vi "Main_12b-2.vi"() -> ()   [LabVIEW 2023]
uses:
  ENUM_Type.ctl
  <vilib>/Utility/error.llb/Trim Whitespace One-Sided.vi
panel:
  out "Fit Array":i32[](array[numeric])
  out "Stream array":T1[](array[typedef])
  out "Rows Left":i32
  out "Answer":u64
  in  "Puzzle":string="??#.????#???.#?# 1,5,1,1,1\n?##?##??#? 7,1\n??????#???. 1,7\n??#?#??#.?#.??#? 5,1,1,2\n???????.??? 1,3\n?#..##?##??###??#? 2,13\n?.????????.???????? 1,5,1,6\n?.???#???. 2,2\n??#..#???#? 1,1,4\n?.?##?????#??? 1,5,2,1\n.???#?????##??#.? 3,8\n?????????????.#.. 4,3,1\n..#???????.? 4,3,1\n????#??.?.#??? 7,3\n#??#???##??.?? 4,1,3,2\n??#?#?##?.???#??. 6,5\n???.#??.??###?.#?? 3,1,5,2\n?.????##??#?? 6,3\n???..?##????.? 2,3,1\n?.?#????.??#?#.? 1,2,1,3,1\n?.?###.???? 4,2\n?#???..??##? 4,3\n???#????#?. 1,2,3\n#???#???#??#???.? 1,10,1\n???????????????????? 1,5,6,3\n???????#??? 2,6\n??.??.????.?#?????# 1,1,2,1,4,3\n???#???.??#? 1,4,1,1\n???#???##??##? 3,2,3\n????.??????#?.#? 1,1,1,4,2\n?.#??#???? 1,1,5\n??##???#?.##??..? 4,2,4\n??????#.????.# 4,2,1,1\n??????#??#?.??? 2,7,1\n.????????##.?.?.##? 5,2,1,1,2\n.??????????#?#. 3,1,2,1\n?????????????. 2,1,5\n?##????#?.?????.#??? 2,1,2,3,3\n?????????#?.?????#? 1,2,1,3,4,2\n..?.#???.?##.? 1,3,2\n.??????????????? 10,2\n?.?#????#?.??? 1,1,2,2\n??????.#??.?.? 1,1,1\n#???#?#??#????? 1,2,1,5\n???.?.??#????.? 3,6\n.#.???###???.#?..??? 1,8,2,2\n.???.??#????# 2,4,1\n.????#?#?? 3,3,1\n?###??#??## 4,2,2\n??#?#???#???.??. 3,5,1\n???####??##..?#.#.?? 9,2,1,1\n??#?#???#.?. 5,1\n???#????#???##?# 2,3,3,1\n?#???????#???#??? 1,3,3,3,1\n#???#????#.##..? 8,1,2\n?????.?#?#??? 1,5\n.??#.??#?.? 1,1,1\n?#?#???#???.??? 1,1,4,1,3\n.????#.?.#??? 1,1,2,1\n.??#?.??#? 4,2\n#????????. 1,4,1\n??.#?#????#?...?? 1,8,2\n?#.#?#.??##? 2,3,1,2\n...??.?#?? 1,1\n?.?.????#..? 1,2,1\n?##????????.??.?#??? 6,1,1,4\n?.??#.??.?.???? 3,2\n.????.?????.???.?? 4,1,1,3,1\n?????????##???????#? 2,1,1,2,2,2\n???.?????.????? 2,3,5\n???#??????.??#??.? 1,6,1,1,1\n??##??????###??? 12,1\n?.??.?????? 1,1,2\n??#??????#?.. 2,5\n???#####????. 1,8\n.?#?##??????#??.???? 6,2,1\n?.#??#???????#????? 1,1,12,1\n??????????#.?..?##? 1,1,1,1,3,3\n???????#???.??## 10,4\n.?#????.?.???..? 1,1,2\n.???#?#????? 2,2,1\n#????#?.????##?#?# 1,5,1,5,1\n???.##??????##??#? 1,2,8,2\n??#????????????#? 6,7\n????.??.#.?#?#? 1,1,1,1,4\n??##?#??.#???? 6,1,4\n?#?.?#????????#?. 3,2,4,3\n..??????##?# 2,1,2,1\n?????????.???? 4,1,1,1\n.??#?????.?.?. 1,6,1\n#.?#?#??????#??# 1,6,2,1,1\n.#?.#.##??# 1,1,5\n??#?????#?????? 5,4\n.#??.?.?.? 2,1\n.?#???##.????##?? 7,2\n?#?.??????#??????# 1,8,3\n?.#??#??.?#.. 4,1,1\n?#?#?#??????? 7,1,1\n?#???????? 6,1\n????#..?#???##? 1,1,2,3\n..?????#?###??.? 1,9,1\n?##???.???#?# 4,4\n??.??#???..??#? 1,2,1,3\n#?#??????.??#?? 8,1,3\n???#?##?#?? 2,6\n.?.???#???.#?????? 1,3,1,5,1\n?#.???????# 2,2,1\n?.???.??.? 1,1,1\n?#?#?#??????#??#??? 1,5,2,4,2\n?#??.?#?????.?#. 4,6,2\n#???.?#?#??#?.??#? 2,7,1\n.??#...???????. 3,1,1\n?..???##??. 1,6\n??#??#?#??? 2,4\n?.?.??.??????#?. 1,7\n?.?????????.??. 2,2,2\n???.?????? 2,1\n???.??????????? 1,3,4,1\n?#????#???#??? 10,1\n??#???.?????#???# 6,3,1\n????.?##??#??# 3,8\n?????????????. 1,7,1\n?..?????.#???.. 1,4,2\n?.???#???#? 1,5,1\n#???.????? 2,1,1\n?#.??#?.???? 1,1,1,1\n????.?#???.???. 1,1,4,2\n.?#??#??.??????? 2,4,6\n.??.?##.??#?#.??? 2,3,2,1,1\n..??????#?.?? 2,2\n???#?#??.##. 3,2,2\n?..?????????##?#??? 1,13,1\n??#?????#?.??#?????? 6,2,5,2\n???.???#???# 1,1,3,1\n??##????.?. 4,1\n??#??#??#?. 3,6\n.??????#????#.#.?? 1,1,8,1,1\n?#?#?.?.?.###??#???? 5,1,1,3,1,1\n???.#?#???.?? 1,1,5,1\n?????####??????? 2,5,2,1\n????.??#??#? 1,1,2,1\n??.?????#?#.????? 2,3,3\n?#??#?#?.????.??? 2,3,2,2\n?????????#??.??????. 1,6,1,1,1,1\n???.##?##??#? 1,6,1\n????#?.??.. 4,1\n?#??#?#???.????#?# 4,4,6\n?????#??#.#? 1,2,2,1\n?#?#?#??###??? 1,1,7\n.##?.????? 3,3\n??#???###????? 1,6\n.?###????????##?#?? 7,1,5\n..?#????????#? 3,5\n#?#???.??? 1,1,1\n#???????????#??.??? 10,3,1\n???##??#??#?.?????. 10,3\n?#?????.???????## 3,2,5,3\n??.??#####???. 2,8\n???.?????? 1,1,3\n???#???????????. 6,4\n#???#?????##???.?#? 2,1,1,5,2\n?#?..???#??????. 2,7,2\n?????##?#? 2,3,2\n.#?..????# 2,3\n???????#??#.?..??.. 3,1,1,2,1,1\n?.#??#????? 1,3,2\n???..?.?.? 1,1,1\n?#.?#??#???.##.? 1,1,4,2\n???#?#.??#??? 4,1\n??????#????.???? 6,1,1,1,2\n???..??.#???? 1,1,1,2\n????????.? 1,1,1\n?..#??.??. 3,1\n?##.??#??? 2,1,1\n?????#?????#?#?? 2,12\n?#??????#???.?? 1,6,2,1\n#??.???.??##???.#? 2,3,7,2\n???????..????#????? 2,1,1,7,1\n????#??.?????? 1,2,4\n?###?#?##?##??.??. 12,1\n?#??#.?.??#?... 3,1,1,1,2\n??#??#??#????#? 9,2\n???????##????? 1,1,5\n?.?#????#?.??.?? 3,3,1,1\n???..??????#..??#? 1,1,7,1,1\n??.???###???#..? 1,1,5,1,1\n??.??.#????#????# 2,1,7,2\n??????#?#??????# 1,6,1\n#?.?...??.??????? 1,1,1,6\n??#?##??#?..## 7,2\n?#?###..?.#?##??.?.# 5,6,1\n.??.?.???. 2,1,1\n?.???..?.?#?.??.???? 1,3\n.#?.??????.?.?#??? 2,6,4\n???##...??. 3,1\n????????????#?????. 4,6\n????#.??#? 1,1,1\n?.?#.??..??#?????..? 1,2,1,8\n?????.??.? 1,2,1\n??????##?.?? 1,4\n???.????#??? 1,1,5\n.??#???.#.#??#??. 6,1,2,1,1\n?.????#??##?????? 1,1,1,7\n??????##.??? 3,2,1\n?.????#?????.?.? 1,4,2,1\n?????????????## 1,1,2,4\n.?##??#??.??# 4,1,3\n??#?##??#?? 2,5,1\n?????.###??.?.#??# 1,1,4,1,1,1\n.????????##?#? 1,7\n??????????.? 7,1\n.?????###????..#. 12,1\n????.????? 3,1,1\n#.??#????#????#????? 1,5,1,7,1\n.##??????.??##? 7,3\n?..?.???#?????###? 1,1,5,5\n??????#???. 1,1,3\n??.#???????##????. 1,2,3,6\n?.?.?.?.#???????#?. 1,1,1,1,2,7\n?????#????????. 1,1,1,4,1\n?.??#??#?? 1,1,2\n??#???.#.?#?#?? 1,1,1,1,5\n?????????.? 4,1\n??.?????#?.?.#?? 7,1\n??.?#.?????#??. 2,7\n?????##..? 1,4\n?????????. 4,1\n??.?..?#???? 2,3,2\n????.####??###? 2,4,4\n?####???##??????? 10,1,1\n???#?#???# 1,5,1\n????###.??.?????#??. 6,1,6\n#???????#?. 2,1,4\n?#?.???##???????#? 3,1,2,1,6\n???#??#?.?.?????? 1,5,1,1,4\n?.#???##???.?.## 1,3,2,2\n???..##?.?.? 2,2,1\n?.#?#?????. 3,1\n????.##?#?#??##?? 3,12\n#?##???????? 1,3,3,1\n???.#?.????##? 1,2,1,4\n???.??#???? 1,3\n.???###??.???????# 7,5,1\n?#.??.?#???##?. 1,1,1,4\n.????###????? 2,6\n???#???.???????#?? 1,2,1,3,4,1\n.?.?????????? 3,5\n??#???#?.###????.?? 7,3,1,1,1\n#??###??#?#.????? 11,1\n#.?????#??#.##???.? 1,1,7,5\n??????.????#???? 1,1,4,1,1\n?.?#?#?#??###?? 7,4\n????#???#?#?###????? 1,2,10,1\n????#????? 1,4,2\n???.#??#????.?#??.?. 3,2,1,1,4,1\n?????.?#??????. 1,2,1,1,1\n?#???????#?#?#???.? 2,12\n?#??..??.???###?? 4,2,1,5\n##????????#.? 5,2\n#?#?.?.??###??#?. 4,8\n??##?.???? 3,4\n?.????##???????? 8,1,1\n#????#??#???#?#.??? 15,1\n?.?????.#? 4,2\n?.##???..?? 1,3,1\n#????#??????????#?? 2,7,2,3\n???.????#? 1,1,2\n??..#?????### 1,3\n????????.?? 2,4,1\n#??##??#.?????.??? 1,5,2,1,1,1\n???#.?#?#?. 3,1,2\n?##?#??????#?#.# 3,3,3,1,1\n??.#?..??? 1,1,1\n?#??.???#? 1,1,3\n???#???????.??##?? 8,3\n??.#.?#???#??.? 2,1,7\n??????.####?.?#?# 4,4,4\n??????????? 2,2,1\n?#?.??.???.? 2,2\n????#?#?## 6,2\n.??###??????.? 5,3\n.???#.#????? 3,5\n?##?#?.?#?#??. 6,2,1,1\n#.???.??#?####?..? 1,1,1,8,1\n????#???#???# 1,1,2,3\n?????.??.#???#? 3,5\n?#??..?????????#?. 1,1,3,1,4\n#?????????????.?? 6,1,1,1\n?#?????..?????#??# 3,1,1,5\n???????.???????????? 1,4,1,9\n.????????????.. 2,1,6\n.?#??????. 2,4\n??#??#???#.???#? 1,5,2,1,2\n.?.???????.?.#??? 4,1,2\n##?.??##?..???. 3,4,3\n??..??#??#?. 1,6\n??#??????????##???? 2,6,4,1\n??..????##?????? 1,5\n##????????.??.#??? 2,6,4\n?#??#...?????# 2,2,1,2\n?..??????.???.?# 1,1,3,1,1\n.?###??#???#???? 7,4,1\n?#?.?????. 2,2\n??..????.?????# 1,1,2,2\n??##.#??????.##??#?? 1,2,1,1,1,5\n??.##??????#???#??? 4,8\n??#?????????. 4,3,2\n#????.???? 1,1,1\n?..??.?????? 2,3\n??????#??###???? 1,1,9,1\n?????#?#???????.. 1,6,3\n?#??.???#?##. 3,3,2\n?..##?#???????#?? 9,1\n???.?#?#?#?. 1,5\n???##?#???#?# 8,3\n?##??#??.??.???????? 2,3,1,6\n.??...?????????#.#? 1,6,2,2\n????.#??#?#.##?. 1,1,1,3,3\n?#?#?????.??????. 5,3\n??.????##???. 1,5\n????#?.???? 2,1\n????..??#???. 4,2,1\n???????.?# 2,1\n????????????? 1,1,3\n???##??????###.?#? 2,2,2,3,1\n??????#?#?#?#?## 3,10\n?????#??..????????? 8,5\n??##???????.??? 6,1,1,2\n?.???.????.??? 3,1,1,3\n.?.???.??? 1,2\n.???###???#??.?? 5,1,1,1\n????#?.##?###.# 1,3,2,3,1\n.?#???????? 1,4\n?#?#?????????### 8,6\n?????..???.???? 4,3,1,1\n..?#?.?#??? 1,5\n.????.??#? 3,3\n?##????.?#??????..?? 7,3,3,1\n?????##??.?.??...?? 9,2,2\n??..#??####??.?.?#? 8,2\n??????##????? 1,1,6\n??????#??.???#? 7,5\n???#..??.????. 4,1,2\n.#?.?###??? 1,4\n????###?...?#?#? 8,4\n?????#???#??????? 1,1,6,1,1\n.??#?#?##??????? 7,1,1\n.#.?????#.?#### 1,2,1,1,5\n?#??..#??.#?? 3,1,1,1\n????#??.???. 3,1,3\n#.???#???. 1,2\n???.???##.???.? 1,1,2,2\n?#?#..?#????##?.?. 3,9\n.?.??.????? 2,2\n??????.?.##?#?.? 5,4\n???#???.????? 7,1\n??####?????.???#?? 6,3,4\n?.?...?#.#?#??? 1,2,5\n??.??#??#?#?#??.?? 2,3,7,1\n?#?.???????? 1,1,1\n????????#?##?#??? 1,2,9,1\n#???.???#????.??#??? 3,1,1,1,4,1\n.??#?.?.#??? 2,1,2,1\n.?##?###.###?#?.??. 6,5,2\n.?.???????#????##? 3,10\n?.##???..#? 5,2\n????????????#??.???? 1,1,10,1\n??##??#.??#??#?? 5,3,2,1\n?#???#.??????..# 6,4,1,1\n????????.? 1,2,2\n?????#??#??#????#??? 14,2,1\n???#??.???#?#???? 4,7,1\n.?.##?.???#??..????? 1,3,4,2\n??????#??????? 1,1\n..#?##??.????. 5,3\n??????????#.? 4,1\n#????.???.? 1,1\n.?..?#.??? 2,1\n?#.??##??.##?.?? 2,4,2,2\n??#????#??????? 9,1\n.#?.##?##.#???? 1,5,1,1\n?#?###???#??#?.??? 11,1,1\n???#??..?? 3,1\n#?#??????#?????#? 12,2\n??#?#?.???.? 2,2,3,1\n?#???.?.??#?#???? 5,1,8\n.???#?#??#?????. 10,1\n??????.?????.? 5,1,1,1\n.?.??????????# 3,7\n.#?.??..##??.?#..#? 1,1,4,2,1\n?##?#??.??###?????# 2,1,1,1,7,1\n?##?.???.? 2,1,1\n?????#.#?##.?#? 1,1,4,1\n?#?.??.?#.#.##.? 2,1,1,1,2\n???????.#.??##??.?. 6,1,3,1,1\n.?#??#???????#???.#. 3,1,1,2,4,1\n?????#?.##??##??.?? 1,2,2,3,2\n#??.???????? 1,1,1,1\n????#?.##?.?#?#?# 5,2,5\n.?.??.#?????????..?# 1,1,6,1,2\n???#?#?????. 7,2\n???????##??#?.?#?.? 1,8,3\n.?..?#?#???? 4,1\n??.?#??.????. 1,1,3\n????##???##???#??? 12,4\n?###?#??..#?.??? 6,1,2,1\n##??..##?#????# 3,2,1,1\n?????#?##??##???#?? 2,13\n#?..???##???##?#???? 2,6,4,1,1\n.????.?....#????. 1,3\n?.?.??#??#.?# 1,2,1,2\n???#??.??#.? 1,1,1,2\n.????#?#???#??????? 12,1,1\n?..#??#?##??#???? 1,1,2,3,5\n.#??##?##??????.?# 2,11,2\n.?.#?#?.?#???#.? 1,4,6\n?#.##??.????? 2,4,4\n???.??????.??. 2,1,1,2\n???????.?##.#???.? 1,1,1,2,3,1\n??..???????#?.? 5,2\n?????#????? 3,2,2\n.##????..#??.. 6,2\n????.??????.???###? 3,3,1,5\n??????#?.???# 1,3,1,1\n????#????. 6,1\n??.?#????. 1,4\n??????#???##???. 6,1,3,1\n?.?#.????. 1,1,4\n?##??.#?#??.#?? 3,1,1,1,1\n?.?#??????. 1,5,1\n???????#?. 1,4\n???#????#?##?#?????? 2,2,1,1,6,1\n??##.?????##??#.? 1,2,7,1\n????????.# 4,1\n.???#????? 1,1,1\n?.?#??.????.?#?? 1,4,2,2,1\n.?##?#???.??..?#? 3,3,3\n?#??.?.?#??? 1,1,4\n????..#????#.?? 1,1,1,3,2\n???#?..??? 5,1\n?##???##.?. 3,2,1\n??#???.???### 2,1,1,3\n????.?#??##?. 2,2,2\n?#???##??#?????#.??? 2,11,1\n???#??..?##??# 5,6\n????.??#???.#?#.?#?# 2,5,1,1,1,1\n?.??????#??? 2,3,2\n#.#???..????????. 1,1,2,6,1\n?.?..?.#??????##?? 1,1,1,1,3,5\n.??.?.???? 1,1,4\n#??#.?#?#???#??????# 1,1,2,1,1,8\n?????.?#..#. 3,1,1\n????##???.?????.. 5,3\n.????#???????? 1,5,1,1\n##?..#.???#?????? 3,1,1,2,1\n#??##???????????. 1,11,1\n????????#. 2,1,2\n.#?#?????????. 1,4,2,1\n#??#??.????????????. 5,5,2\n..?#?#???#???????.?. 9,1,1,1\n?#?.?????????... 1,6\n??###??#?#?.? 5,2,1,1\n.?????????.??... 6,1\n?.?.#??#??????#?#. 1,2,7\n??.?#?.#??.??. 1,2,2,2\n?##?#.?#?. 3,1,1\n??.??####???... 2,6\n.?????#????..?..??## 7,1,3\n.#?##???.? 5,1\n?.?.???#.???. 1,1,2,1\n?????.???## 1,3,2\n.????#??.??.?. 5,1\n.?#??.???? 2,4\n??#?.??#?? 2,2\n?.??.??????.?????? 1,1,2,1,1,5\n?????#??????.??? 1,5,2\n#..?#??.?# 1,2,1\n???????#???#?#???.? 5,8\n??.?#??#?? 1,2\n????#.#??#? 3,1,1\n#?#?..?..?????#??? 4,1,2\n??????.?##?##.??? 1,4,6,1\n?.????###??? 1,8\n??##???????##?????. 8,4,1\n?#.?#.?.?????? 1,1,1,6\n???#?.?.#??##???##? 2,10\n.?????#?.?##????#?# 1,3,2,5\n#?.?.?#?..???#? 2,1,1,2,2\n..???#??.??#?? 5,3\n.????##??? 7,1\n??#?###???# 7,1\n?????????????????. 10,5\n??#?#?????????###?? 3,1,1,1,4,1\n????##???.#??? 1,6,1,1\n.##??????##?..??#?## 11,2,2\n?#.????????? 2,1,1,2\n??????#?.??#??..???. 3,1,5,3\n.?##??????????#???? 3,1,1,1,2,1\n?#?...?#?????#?.? 2,8\n###?#.#?#?????.#???? 5,1,2,2,4\n?.???#?#.?????#?.? 6,5\n#????#???#???#?#? 2,2,3,3\n??#??.??#.?#? 2,1,1,2\n##.?...????????#?#? 2,9\n??#?#???#???? 4,1,1,1\n.???#?.?????.?#?.#. 4,1,1,1,1\n??#.?????#?????##? 1,1,1,7\n#???????#?????#? 1,1,8\n????##?#?#??##???#?. 1,8,6\n#.???.?????.#?? 1,1,2,3\n##?????#??.????#? 2,1,3,6\n#???###?##.? 1,4,2\n#..??????#???.. 1,10\n?????#???.?#?#??# 7,7\n???.#????#?????.#? 1,1,1,6,1,1\n??.#?#?????????.?# 1,4,2,2,1\n?#?#?..?#? 1,2,2\n?.?##.???###?? 3,5\n.?#????#??..?? 2,5\n???#.#??.?.????..#?? 2,3,4,1,1\n???#..?????.? 1,1,5,1\n?##?#??????##? 4,1,5\n??#.#?###?##?????#? 1,1,8,1,1\n.#?#??#.#?.? 1,1,1,1\n????????#?#?##??# 5,1,1,5\n.??#?.?#?????.?????? 3,7,4\n?#?????#.?#? 2,5,2\n????.?#????#?????#? 1,9,2\n?#????#???.??.??.. 7,2,2\n?#.##???????.?#.? 2,5,1,2,1\n?.##?#?.????#?#??. 2,1,6\n?###??#.#????##.?? 5,1,1,1,3,1\n.??#?????#???#?.# 3,1,2,2,1\n?.????.??.#?????? 1,3,1,5,1\n????##?##?? 6,3\n.?#???.?.????? 2,1,4\n?????...??.. 1,1\n??#????..??# 1,2,2,3\n?###.?????#.???#? 4,3,1,2\n???##????.?#.?#??? 1,2,2,2,5\n?#.?????.?###?##??.? 2,5,6,1,1\n.????.??.?????????? 3,10\n??.?#?#.#..??? 1,3,1,1\n?.?#?#??.?. 5,1\n???#.?????##???#??? 2,13\n??#???#.#???#???#?? 2,2,11\n?#???????? 4,1\n??????##???##????# 2,10,1\n???#????#?? 3,1\n##????#.?.? 3,2\n.????#?????? 6,1\n?.??.????#? 1,4\n?????????.? 1,4\n#?#??#?##????#????#? 14,3\n#..#????#??? 1,1,4,1\n.?.##????.?? 1,2,1,2\n???.#??#?#?.?????? 1,1,7,1,1,1\n..?#????.#???##????? 3,2,7\n?????.??.? 3,1\n.?#??#?#..?#?.?##.?? 2,4,2,3,1\n???#?????.# 8,1\n????..##?.??#? 1,2,3\n.?????.?#? 1,1,1\n??#?.#?#?#?.###?. 1,5,4\n???.#????##.???##? 1,3,3,5\n?????????#?#?????? 7,2,1,1,1\n#.?##.???.?#?..?.#. 1,2,1,2,1,1\n???#.???.?? 1,1,3\n??.?.??###??.????.? 1,1,7,1,1,1\n.?.#.?#?##?.???# 1,1,5,1,1\n???###?#???# 8,2\n?.????.#..##??? 1,1,2,1,4\n??#????####???#?. 3,8\n#..?#????##?#?. 1,3,3,2\n###.??.##.? 3,1,2\n???##?.????#?#??? 4,5\n?.??.?.?.??? 1,1,1,1\n.#???##??#???##???? 1,1,5,4,1,1\n?..##..??#...?.?.?? 2,1\n?#..#???.?.??# 2,2,1,1\n????#?.#??.? 1,3,1,1\n?#?????#???.????? 3,3,1,2\n#.????###???.?#???? 1,7,2,2,2\n?????.?????? 3,1\n.??#???????. 3,1\n?.?#??.?#???##?#?? 1,1,1,11\n?#????#?#. 4,1,1\n..#?###???#.??? 1,7,2\n#....????? 1,1,1\n?.????????.? 4,1\n##?.??????.#??? 3,2,1,1,1\n?????.?#.?????#??.. 2,3\n?#??##?#?#?.??##? 7,2,3\n.?.?????##.??? 1,2\n.#?##?##?.?????.?#.. 7,1,1,2\n???..???#?. 1,1,2\n...?.???#?#? 1,4\n?????#????#.? 7,2\n??#????##???##. 3,2,4\n???.???????. 2,1,1,1\n###?..?????.. 3,4\n.???????????..?. 4,2,1\n?.?.#??.?? 1,1,1\n?????????????#?? 6,6\n..#?????.??? 4,1\n???#??#?##.?#?.?? 7,3\n#???###??????#?? 1,1,3,2,3\n?##??.??#??????#???# 3,9,1\n???#??#??.??????#??? 7,3,1\n.???###??##?#.?.??? 6,2,1,2\n?.?#?#?.?.?#? 3,2\n.??#.?###???##?? 2,5,3\n????.?????#??###?? 3,12\n?#?##?#..#??#?? 5,1,1,2\n??#??...???#?#???. 1,7\n???##???.???#.?. 7,3\n??.#???#.# 1,5,1\n??###???????????# 5,4,3\n#??..#??##.?????.? 1,1,5,2,1,1\n????#.???#????.. 3,4\n#?????.#??? 3,2,3\n?#?.???????. 2,2,2\n?.?????????## 1,1,4,3\n#????????..#?#????? 3,1,1,3,4\n???#??#??????????.. 7,1,1,2\n?##.??###???#?#??# 2,1,3,1,3,1\n?#?.???#?#?#?.??# 3,5,2\n??#????.??#?#? 3,3,4\n###?##???#?#??.?.# 8,3,1,1\n.??.?#???#??? 2,1,3\n.???#??###?? 1,6\n???????.???????? 7,1,2,1\n.??###?.??#.? 5,3\n?#???#???????#?#???? 2,5,1,4,2\n????.?????#?????? 1,1,7\n.??.?.?#?##?#???#?? 1,11\n?????#???? 5,2\n?.??.???.#?? 1,1,3\n????#???????? 5,3,1\n#?##????#???#?.?#.# 4,3,1,1,1\n??#??????#?? 1,1,1,4\n.????.#?????#?? 1,2,1,1,3\n????????????????? 1,4,3,2\n????.#?.##?##?#?#?? 3,1,5,3\n??#?###??? 1,3,1\n????#???....? 8,1\n.????.???.???..???. 2,3\n?????.??#? 4,2\n#??.#.????#.???###? 2,1,1,1,1,4\n.???????.??????# 6,5,1\n??#??#?????.??#. 1,4,1,2\n??#?.??.??????#?#??? 4,1,3,1,5\n?#??#???????#..??? 4,7,1\n???#?##?????.?? 5,2,1\n.?###?????#?##??. 6,7\n#??#..??????#?? 1,1,7\n.??#?#??????# 4,1,2\n.###??####????#???# 4,13\n????#?????.?. 6,1\n#?##???#????? 5,1,2\n??#?.##??????????? 4,4,5,1\n.????#???? 2,1,3\n?.?#.???????#?.????. 2,4,1,1,3\n?.?#?????##??????? 2,10,2\n?????..???##? 2,3\n?#.#.???#???.? 1,1,1,4\n.?##???##?????###??? 15,2\n?#.#?.????.??.?#?.? 1,2,3,1,1,1\n????#??????. 5,1\n?.#.????##??.?. 1,7\n??.?#?..??#?????.? 2,6\n???##?.#?.?#? 3,2,2\n?#?.???.?? 1,2\n?????????..?#??? 1,1,2,2,1\n?#.??..??? 1,1,2\n??.????##???? 1,1,3,1\n??####??????#.?.??? 5,1,1,1,1,1\n.??#????.?# 2,1,2\n..#?#???##???.?.??# 1,1,4,1,3\n??.##..??. 1,2,2\n?#???#?????? 2,5\n????##?#?.???.? 5,1\n.?#?..????#??.??? 1,4,1\n.#####??????#??. 7,5\n???.?.?.##?#???. 1,5\n????###??.????#?? 8,5\n?????#.???#?.?.?# 4,4,1,1\n????????.?###????#? 1,3,4,1,3\n?.?????.?#?????# 1,3,1,2,1\n??.??????????? 1,3,1,1\n???.?????#??? 1,6\n?##???#?#????#????#. 3,3,3,2\n??#?.?.???### 2,1,3\n#??..?##??????.??? 1,1,3,1,1,1\n???#??.?.#???#? 6,1,2\n?#?..????? 3,2\n?##??#???? 5,2\n??.??????.?#? 1,4,2\n.#?##???.???#??????? 7,4,1\n?.#???..????? 4,3\n.???..?#??##?? 1,7\n.#???????.??? 1,1,1,2\n?#?#???????##. 6,3\n#.?.#?????#??#?#???. 1,1,1,6,4,1\n.???????.?#?#??????? 2,5\n??.?.?????? 2,3\n???.????..#? 1,1,1,2\n??#??.?#?..???##??## 2,3,8\n#??.?.?#??#?. 2,5\n?.????.????????? 1,2,3,1,1\n???.??.??????????#. 1,1,1,3,3\n???????.??? 1,1\n##??#????????.?????# 2,2,6,1,3\n??.?????##????## 2,1,1,8\n???.??#?????#??.. 1,3,6\n??#?#??#???????.? 7,1\n.?#.????#??#? 2,4,2\n?????.??#.??? 1,2,2,1\n??##???.????????. 6,6\n..???..?.?.? 3,1\n??#?.??????.. 2,1\n???????##?????. 1,1,4,2,1\n??##..??#???. 2,4\n?????#??????#? 1,2,4\n..??#???#?????#?? 3,2,5\n???.??#??.???#?#??? 2,5,6,1\n?#?#.??##.?. 3,3\n#??#.?????.?? 4,2,1\n?#???.?#???#???.. 4,9\n????.??????#?#??# 2,7\n??#.??????????????? 3,7,5\n??#????###? 1,4\n???#????#.#.??.. 1,3,2,1,1\n???#?.???? 1,2\n?.??.?#??? 1,3\n??.????#??#.?.? 1,2,1,1,1\n..??????.?? 4,1\n??#?.???.???? 3,1,1,2\n?.????#????#? 4,3\n?#?????????????? 5,4,1,1\n?..?????#? 1,1,1\n?.?#???.?? 4,1\n#??#.????? 4,4\n#??.?????????????? 2,1,1,3,2,2\n.???#????.?? 1,1,2,1\n??.?##?.??#??#?#??.. 4,10\n????##????#???#.???? 2,3,2,1,1,1\n????????.??###?????? 7,5,2\n????.?.#??? 2,1,1\n.#?..?#????#???## 1,12\n#???##??.???????? 1,5,2,1,3\n???#???#?.#??..? 7,1\n?#????.???.?#? 6,2,1\n.#?????????#???. 6,1,3\n???###????????#?#?#? 8,2,1,4\n?#?#..??#???. 4,1,3\n.???##?#.??? 1,4,1\n??????????? 5,1,1\n??.#?#.???? 1,3,3\n.#.###??????.#? 1,4,1,1,1\n???#??.?.????? 1,3,4\n?#.#????????????# 1,1,1,8,1\n.??????###? 3,3\n.#???????#???? 3,1,4,1\n??#??.?#???#...? 3,6\n?#???????.?#???.???? 9,4,1,2\n???#.??#??? 4,3\n??#????#?#.??.?# 1,3,4,2\n????#?##?.??????? 6,1,2\n.??##?#?###..#??.?? 3,5,2\n??###???##?#?.??. 12,1\n?..#?????#????#?# 2,1,2,4\n????###?.?#??#??#. 8,6,1\n????##?#????# 10,1\n#?##?..?##?? 5,3\n?#.?#??#???????? 1,7,2,2\n.#?..?#?#??#. 2,6\n#??#????.??#?#. 7,3,1\n.?.??.????. 1,1,3\n?????.???#?#??.?? 1,3,4,1,2\n????????????#??#?? 4,8\n????####?#? 1,7\n?.#????.????#?.?? 1,6\n?#?????#?##?? 3,4\n?#????#????# 9,1\n?##?#?????.??? 6,1,1,1\n???..?##?..?????? 2,2,3\n#.??.??????? 1,1,2,1\n?##???##.?###? 3,2,4\n#?##????#.? 6,1,1\n.????.??###???#? 1,2,5,2\n?.#??.??#???? 1,3,4\n??##????#???#?#??? 4,7\n?#?.???#??##???#?? 1,1,2,8\n???.?#?##????.? 1,7\n#.?##?#?.#.????# 1,5,1,1,3\n#???..??#????#????? 4,5,2,1,1\n???????.???????#? 1,3,1,2,1\n##???????? 3,1\n?#..?.???? 1,1,1\n..??.#???##???#. 1,10\n.?????##?????#????. 7,4,1\n??..#?..#.#.#?. 1,2,1,1,2\n????.?###?#??. 2,8\n????.#?????? 3,6\n??#??#????#.?.?#.??. 10,2,2\n???#??????????? 8,2\n???.????#??..?. 1,5\n.?.??..?#. 1,1,1\n#??###..???#???? 6,1,1\n???###?..#?#??????? 5,7,1\n????#??#??#?#?.??#? 1,1,2,5,3\n????#??.?.?#???#. 7,1,1,1,1\n?##?#?#?.??#?. 6,1\n???????#?#???.# 1,4,1,1,1\n???????##.?# 9,1\n.?????#.???. 1,2,1,2\n#.?#.??#?? 1,1,1\n?##?#?????? 5,4\n?.?##??.#? 4,1\n?????##???.#?.##? 1,5,1,2\n??????.??? 1,1,2\n?.??.?#?#?#.?##??#?? 6,8\n??#???????????.?? 8,1\n#????????###??#??#? 1,2,8,1,2\n#.#???#?#?#.?????#? 1,9,1,1,1\n#.??#???##? 1,7\n?????##?????????#??? 6,1,2,4\n????#?##??????#?#?# 2,4,3,3\n?#?.##????#???? 1,3,2,1\n?.?.??#?.? 1,1,1\n???????#?#???..??? 1,4\n???.?#??##?#?##.#? 2,10,2\n??#?#???..???.??.? 7,1,1\n?????????.#.??????.? 6,2,1,1,3,1\n?#???##????# 2,6,1\n#?###?#??.#??..#.? 7,1,3,1,1\n???.???#???#?? 1,5,1\n??????#??????.???#? 7,4\n#?????#??.???#.? 3,3,1,1\n?.?..??.?##????.? 1,1,3,3\n?##????.???? 7,1,1\n?.?##.?#?#?????? 3,3,2\n?.??.?.??? 2,3\n?##?..????? 3,5\n??####?..?? 4,2\n???.???????????????. 1,7,6\n#???####???.# 8,1,1\n.#.???#?.????.? 1,2,3\n????????????#?????? 2,3,9,1\n#?#??#????????? 1,5,1,1,1\n.?.????.?#.?. 2,1\n????..#??? 1,1,1\n??##?????#???? 4,7\n?##?????.?#? 5,2\n???????###????##?# 3,1,6,2,1\n##?????.???. 4,2,2\n??#??.??#?..# 1,3,1\n????.#???????#?.. 1,10\n####??###????#.???. 5,3,3,3\n?#.?#???.?#? 1,4,3\n#.?#?#???#.#??????? 1,4,2,1,1,1\n??#????#?###???#?# 5,11\n??.???#???#????????? 1,5,3,1,2\n.??????#???####?.#?? 13,3\n.??????#?#?.??.?#? 10,1,2\n??..??##?#??????.??? 10,3\n????#???#####?????.. 10,2\n????#?#??#???###? 3,7\n????.#?.?????#.? 1,2,6\n???????????..? 1,4\n?.???#?????.? 1,2,1,1\n#??#??#?#???#?#.?? 1,8,3,2\n?????###????.???? 1,5,3\n???###?#?##????.??.? 1,9,1,1\n.?#?##???#????##??.. 9,3\n.?.?.?#????????##?. 1,1,1,1,1,4\n?.??.??#????##??##?? 3,6\n??????#?????.#?? 6,1,3\n?#?#???????.?#?.???. 11,3,1,1\n?.?#..#??????.??. 1,1,6,1\n??????#???### 3,8\n???#?#??.??##????#?? 8,1,8\n.#?.??.??#? 1,3\n?????.??????#?????. 2,1,1,10\n??.#????#.? 1,2,1\n???#?????????#?#?? 4,8\n..??..?????.### 1,2,3\n??.???#???.??# 1,7,1,1\n?###??..?.??#??#???? 5,4\n????????#?..?? 2,5,1\n???##?#?????#### 2,2,1,7\n?????#???#? 5,1,1\n??#.?#???####??#??.? 1,11,1\n?#?????##?#?? 5,5\n??.??.?####?. 1,6\n.???????#?????. 1,6,1\n????#.?????.??.?#? 1,1,1,2,1,2\n???.?#?????#.?#?.??? 1,4,1,1,2,3\n.#??????.#?? 1,1,1,1\n..#?.??????????? 2,5\n.??##???????. 3,4\n??#????#??????????.. 1,4,9\n.??#??.#.?# 2,1,1\n??.??????.?#????? 1,4\n#.?#??#???##? 1,2,7\n?###??.#.??. 4,1,1\n???#???#???. 7,1\n?????????#??? 4,4\n???.???????#.? 1,3,2\n?#??????##? 4,1,3\n?#.??.??#?.# 2,2,2,1\n?.#?????.????? 2,1,5\n?.#???#.?#?## 1,1,2,5\n#?#.?##???????#??.# 3,3,1,2,1\n#?#???.?.#.#??# 5,1,1,1,2\n??##?.##?????? 2,7\n.??###?#??#???? 5,1,6\n?.???#?????.?#??? 1,6,2\n??.?.?#??.???.???? 1,1,1,1,3,1\n???.???.###?##???## 1,1,1,6,3\n#???#??##??# 6,2,1\n??##??.##????? 3,7\n?#?#?#?.???##???.?#? 4,1,7,2\n.??#?#????.?##.? 8,2\n.???#???.. 1,1,1\n.????#??.#?#?. 2,4\n#?.?????????..?? 1,1,1,4,1\n?#???#??.? 1,2,1\n#???????????.???.? 4,3,1,1\n????#?#???#???#.?. 12,1\n???.??#.?#???#? 2,1,7\n??#?.#??.?#?. 1,1,2,1\n??#.???#.?? 2,2\n?????#??.????? 7,4\n?#?????????###?????. 1,1,1,1,5,2\n.?#?.#???? 2,3\n???###?#?..??.#?# 2,6,1,1,1\n..#?.???#?#???#??? 1,12\n????##.???? 3,2\n?#?????##?????? 1,2,5,1\n??????#???# 3,1,3\n.##??.???.? 3,1\n???##????...??..??? 6,2\n???????#???. 1,4,1\n?#??#???##?.??.# 10,2,1\n?.?.???#??? 1,1,3\n?#?#?#??..?? 8,1\n??#?.???????#?? 1,10\n?.#???#?#??????? 1,2,4,1,3\n#?#?.?##?????. 4,6\n#?#??.???#? 3,4\n?.?????#?#??. 1,8\n?.?.?.#.??.??#? 1,1,1,1,3\n?#???##??????##???.? 9,4,1\n?#???????????.? 5,1,1\n#???.??#?#????#?#? 2,1,11\n??#???????#???????? 6,1,7,1\n?#???#???????#?. 1,4,1,2\n????#??.???#.?? 6,2,1,1\n???.?#????.# 2,2,1,1\n#???#..??#?#????.? 5,7\n##?#..???.??.#?# 4,1,1,3\n.?..???????.????.?.. 2,3\n.???????.?? 4,1,1\n.?####??#?? 4,1\n??????#????#???? 1,1,6,3\n??#???#.????#??. 6,2,4\n?????????.#?? 5,2,2\n??#??..??????? 3,3\n.#?.??????#???. 1,2,1,1,1\n????????.?#????? 1,1,1,2,2\n?.??.??#??#?? 1,5\n.???#??????# 1,1,5\n?#?????.#?#?????? 2,1,1,3,5\n???#????#????#??#?## 1,1,4,2,5\n?.??.#.????..? 1,3\n??????#?#??? 8,1\n??#??.????#??.? 3,5\n?????#.?????#?#???.. 2,2,6\n????#.???. 1,1,1\n???#?.???#????# 1,2,9\n??#?#???###????#? 1,3,1,8\n#.???##??##? 1,1,2,2\n????#?????.#?.. 5,2\n..????.?????? 3,4\n????.??????? 2,1,2\n.?#??????????.? 7,2\n???#??????#?? 2,2,4,1\n???##?????#??#?. 1,9,2\n#????????.#??.? 1,3,1,1,1\n.??.#???#?##??.?? 1,2,2,4,2\n???.?????#. 1,2,2\n????#????.??? 5,1,1\n.????.??#?#?#???.? 3,5,3,1\n??????##??#.??? 1,2,5,1\n??????##.??.????.? 8,2,1\n?.?.?.?#?#?.????#?. 4,6\n..?????.?#??? 1,1,5\n???#?????????# 1,6,4"
  in  "Example":string="???.### 1,1,3\n.??..??...?##. 1,1,3\n?#?#?#?#?#?#?#? 1,3,1,6\n????.#...#... 4,1,1\n????.######..#####. 1,6,5\n?###???????? 3,2,1"
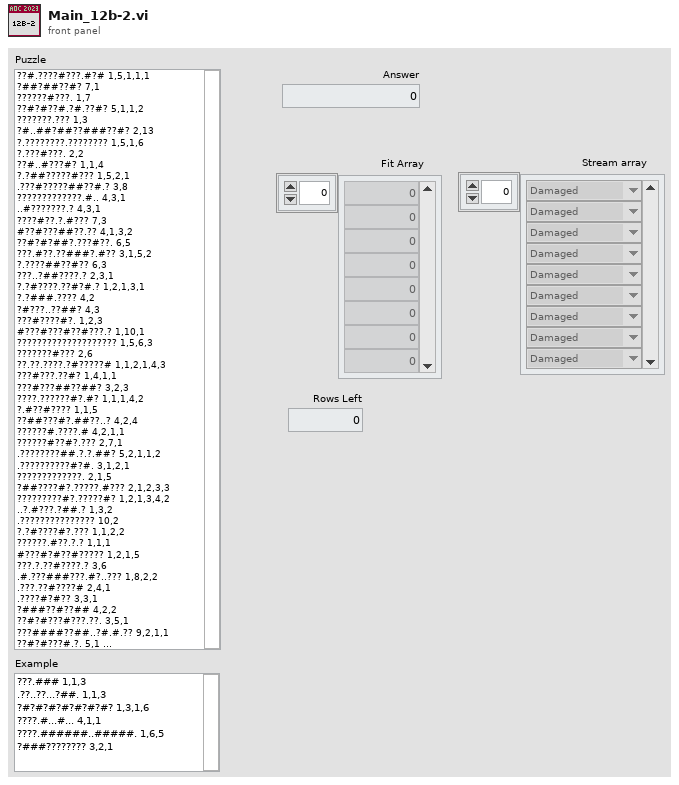
[diagram p1: front panel]
types:
  T1 = typedef "ENUM_Type.ctl" = enum16{"Damaged", "Operational", "Unknown"}
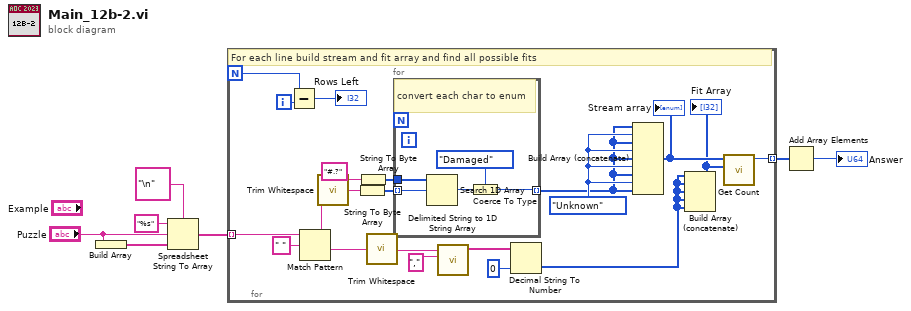
[diagram p0: block diagram]
diagram:
  n1 = Build Array("Puzzle") -> (w7:string[])
  n2 = Spreadsheet String To Array(delimiter (Tab)="\n", format string="%s", spreadsheet string="Puzzle", array type (2D Dbl)=w7) -> (array=w4:string[])
  n3 = for {
    N -> [w13]
    tunnel: w4 -> [w28] mode=indexing
    tunnel: [w8] -> w3 mode=indexing
    i -> [w12]
    w16 = ENUM_Type."Unknown" ("Enum")
    # "For each line build stream and fit array and find all possible fits"
    n4 = Subtract(x=w13, y=w12) -> (x-y=→"Rows Left":i32)
    n5 = Match Pattern(string=w28, regular expression=" ") -> (before substring=w22:string, after substring=w23:string)  [unwired: 1 in, 2 out]
    n6 = call <vilib>:"Trim Whitespace.vi"("string"=w22) -> ("trimmed string"=w21:string)  [unwired: 1 in]
    n7 = String To Byte Array(string=w21) -> (unsigned byte array=w26:u8[])
    n8 = String To Byte Array(string="#.?") -> (unsigned byte array=w24:u8[])
    n9 = call <vilib>:"Trim Whitespace.vi"("string"=w23) -> ("trimmed string"=w20:string)  [unwired: 1 in]
    n10 = for {
      tunnel: w26 -> [w32] mode=indexing
      tunnel: w24 -> [w33]
      tunnel: [w29] -> w15 mode=indexing
      # "convert each char to enum"
      n11 = Search 1D Array(1D array=w33, element=w32) -> (index of element=w31:i32)  [unwired: 1 in]
      n12 = Coerce To Type(0:w31, 1:ENUM_Type."Damaged" ("Enum")) -> (2:w29:T1)
    }
    n13 = call <vilib>:"Delimited String to 1D String Array.vi"("delimiter"=",", "delimited string"=w20) -> ("string array"=w18:string[])  [unwired: 9 in]
    n14 = Decimal String To Number(string=w18, default (0L)=0 ("default (0 I32)")) -> (number=w14:i32[])  [unwired: 1 in, 1 out]
    n15 = Build Array (concatenate)(w15, w16, w15, w16, w15, w16, w15, w16, w15) -> (w10:T1[])
    "Stream array" <- w10
    n16 = Build Array (concatenate)(w14, w14, w14, w14, w14) -> (w9:i32[])
    "Fit Array" <- w9
    n17 = call "Get Count.vi"("Fit Array"=w9, "Stream Array"=w10) -> ("Count Out"=w8:u64)  [unwired: 9 in]
  }
  n18 = Add Array Elements(numeric array=w3) -> (sum=→"Answer":u64)
